vi "tag_factory.vi"(10 "Enum":T1(ring)) -> (2 "Cluster":cluster{"name":string, "text":u32})   [LabVIEW 2021]
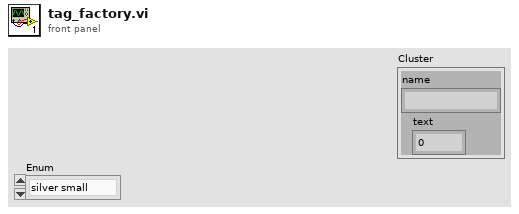
[diagram p1: front panel]
types:
  T1 = enum16{"silver small", "silver medium", "silver huge", "black small", "black medium", "black huge"}
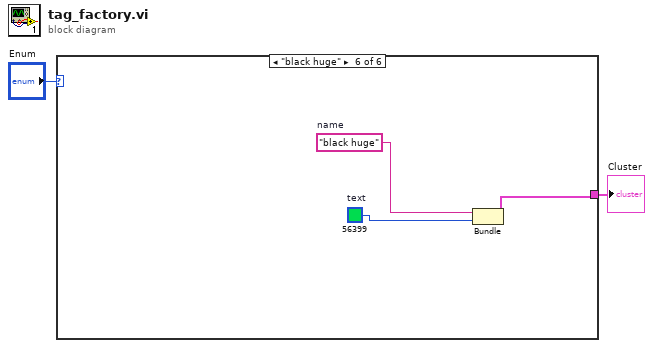
[diagram p0: block diagram]
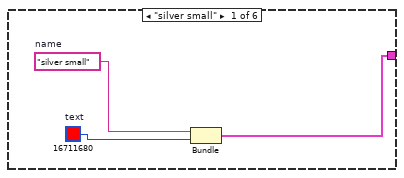
[diagram p2: hidden frame]
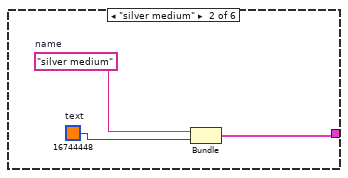
[diagram p3: hidden frame]
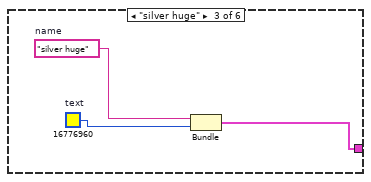
[diagram p4: hidden frame]
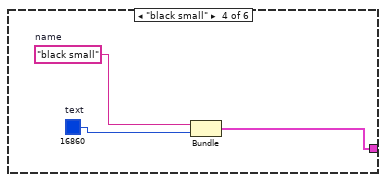
[diagram p5: hidden frame]
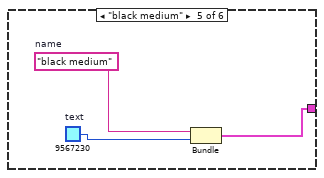
[diagram p6: hidden frame]
diagram:
  n1 = case shown="\"black huge\"" "Enum" {
    tunnel: [w3 w6 w9 w12 w15 w18] -> w1
    frame "silver small" {
      w5 = "silver small"  # name
      w4 = u32 16711680  # text
      n2 = Bundle("name"=w5, "text"=w4) -> (w3:cluster{"name":string, "text":u32})  [unwired: 1 in]
    }
    frame "silver medium" {
      w8 = "silver medium"  # name
      w7 = u32 16744448  # text
      n3 = Bundle("name"=w8, "text"=w7) -> (w6:cluster{"name":string, "text":u32})  [unwired: 1 in]
    }
    frame "silver huge" {
      w11 = "silver huge"  # name
      w10 = u32 16776960  # text
      n4 = Bundle("name"=w11, "text"=w10) -> (w9:cluster{"name":string, "text":u32})  [unwired: 1 in]
    }
    frame "black small" {
      w14 = "black small"  # name
      w13 = u32 16860  # text
      n5 = Bundle("name"=w14, "text"=w13) -> (w12:cluster{"name":string, "text":u32})  [unwired: 1 in]
    }
    frame "black medium" {
      w17 = "black medium"  # name
      w16 = u32 9567230  # text
      n6 = Bundle("name"=w17, "text"=w16) -> (w15:cluster{"name":string, "text":u32})  [unwired: 1 in]
    }
    frame "black huge" {
      w20 = "black huge"  # name
      w19 = u32 56399  # text
      n7 = Bundle("name"=w20, "text"=w19) -> (w18:cluster{"name":string, "text":u32})  [unwired: 1 in]
    }
  }
  "Cluster" <- w1
